vi "Write Index Set.vi"   [LabVIEW 2016, in "CVT.lvlib" / "Current Value Table.lvlib"]
doc: "This VI writes a set of data as defined by the GetIndices function. This VI can provide an order of magnitude increase in performance over a normal index write for sufficiently large data sets. A type mismatch will be indicated by a coersion dot."
uses:
  <vilib>/NI/Current Value Table/Current Value Table.lvlib
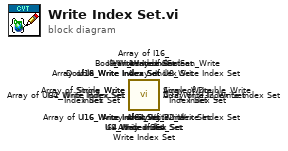
[diagram p0: block diagram]
diagram:
  n1 = call <vilib>:"Array of String_Write Index Set.vi"() -> ()  [unwired: 12 in]
  n2 = call <vilib>:"Array of Boolean_Write Index Set.vi"() -> ()  [unwired: 12 in]
  n3 = call <vilib>:"Array of Single_Write Index Set.vi"() -> ()  [unwired: 12 in]
  n4 = call <vilib>:"Array of Double_Write Index Set.vi"() -> ()  [unwired: 12 in]
  n5 = call <vilib>:"Array of I8_Write Index Set.vi"() -> ()  [unwired: 12 in]
  n6 = call <vilib>:"Array of I16_Write Index Set.vi"() -> ()  [unwired: 12 in]
  n7 = call <vilib>:"Array of I32_Write Index Set.vi"() -> ()  [unwired: 12 in]
  n8 = call <vilib>:"Array of I64_Write Index Set.vi"() -> ()  [unwired: 12 in]
  n9 = call <vilib>:"Array of U64_Write Index Set.vi"() -> ()  [unwired: 12 in]
  n10 = call <vilib>:"Array of U32_Write Index Set.vi"() -> ()  [unwired: 12 in]
  n11 = call <vilib>:"Array of U16_Write Index Set.vi"() -> ()  [unwired: 12 in]
  n12 = call <vilib>:"Array of U8_Write Index Set.vi"() -> ()  [unwired: 12 in]
  n13 = call <vilib>:"Boolean_Write Index Set.vi"() -> ()  [unwired: 12 in]
  n14 = call <vilib>:"String_Write Index Set.vi"() -> ()  [unwired: 12 in]
  n15 = call <vilib>:"U8_Write Index Set.vi"() -> ()  [unwired: 12 in]
  n16 = call <vilib>:"U16_Write Index Set.vi"() -> ()  [unwired: 12 in]
  n17 = call <vilib>:"U32_Write Index Set.vi"() -> ()  [unwired: 12 in]
  n18 = call <vilib>:"U64_Write Index Set.vi"() -> ()  [unwired: 12 in]
  n19 = call <vilib>:"I8_Write Index Set.vi"() -> ()  [unwired: 12 in]
  n20 = call <vilib>:"I16_Write Index Set.vi"() -> ()  [unwired: 12 in]
  n21 = call <vilib>:"I32_Write Index Set.vi"() -> ()  [unwired: 12 in]
  n22 = call <vilib>:"I64_Write Index Set.vi"() -> ()  [unwired: 12 in]
  n23 = call <vilib>:"Single_Write Index Set.vi"() -> ()  [unwired: 12 in]
  n24 = call <vilib>:"Double_Write Index Set.vi"() -> ()  [unwired: 12 in]
